vi "cos_rise_tester.vi"() -> ()   [LabVIEW 2021]
uses:
  <instrlib>/_niInstr/Basic Elements/v1/FPGA/niInstr Basic Elements v1 FPGA.lvlib
panel:
  in  "t":fxp<+/-,16,1>
  out "x .or. y?":bool
  out "Waveform Chart":dbl(graph)
  out "data out":fxp<+/-,16,1>
  in  "change rate":u16
  in  "s":bool
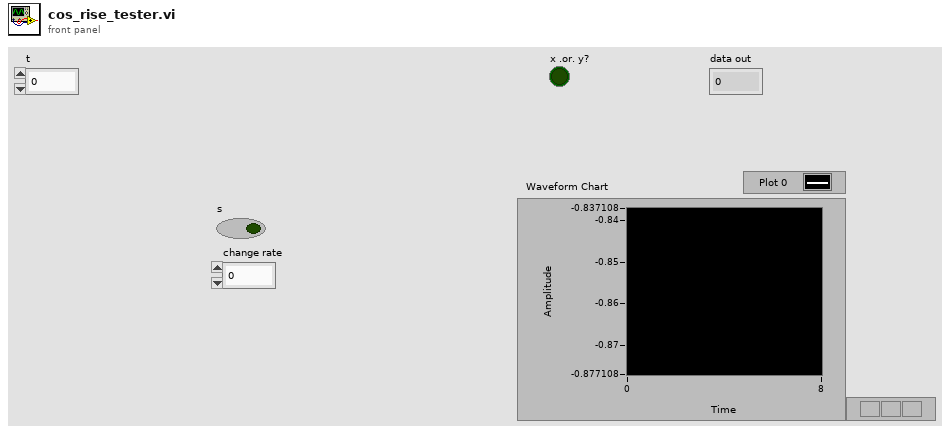
[diagram p1: front panel]
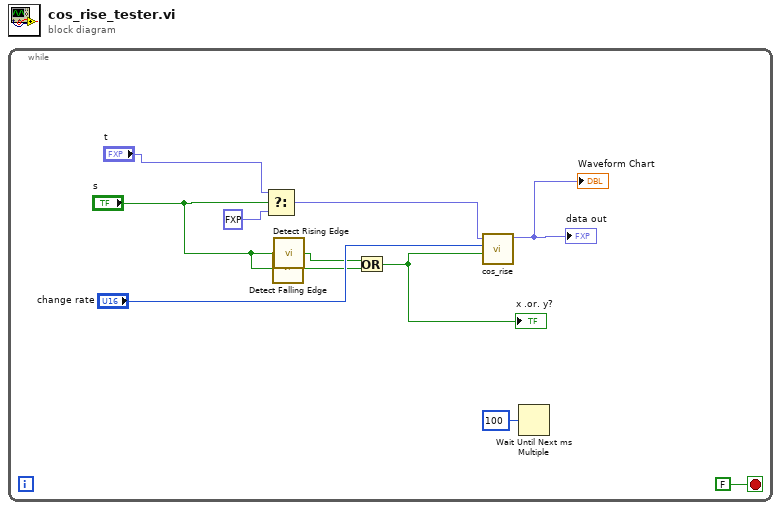
[diagram p0: block diagram]
diagram:
  n1 = while {
    stop <- FALSE stop-if-true
    n2 = Select(t="t", s="s", f=fxp<+/-,16,1> 0.0 ("data out")) -> (s? t:f=w11:fxp<+/-,16,1>)
    n3 = call <instrlib>:"Detect Falling Edge.vi"("signal"="s") -> ("edge detected"=w4:bool)  [unwired: 14 in]
    n4 = call <instrlib>:"Detect Rising Edge.vi"("signal"="s") -> ("edge detected"=w3:bool)  [unwired: 14 in]
    n5 = Or(x=w3, y=w4) -> (x .or. y?=w2:bool)
    "x .or. y?" <- w2
    n6 = call "cos_rise.vi"("new step"=w2, "change rate"="change rate", "data in"=w11) -> ("data out"=→"data out" →"Waveform Chart":fxp<+/-,16,1>)  [unwired: 8 in]
    n7 = Wait Until Next ms Multiple(millisecond multiple=u32 100) -> ()  [unwired: 1 out]
  }
